vi "write time cell with column offset.vi"(5 "Column Relative?":bool, 7 "Header offset":i32, 8 "error in (no error)":errorcluster, 9 "time column offset":i32, 10 "start of last occupied row":cluster{"row":i32, "column":i32}, 11 "NI_report in":refnum<class "NI_report.lvclass">) -> (0 "error out":errorcluster, 3 "NI_report out":refnum<class "NI_report.lvclass">)   [LabVIEW 2016]
uses:
  <vilib>/Utility/NIReport.llb/NI_report.lvclass
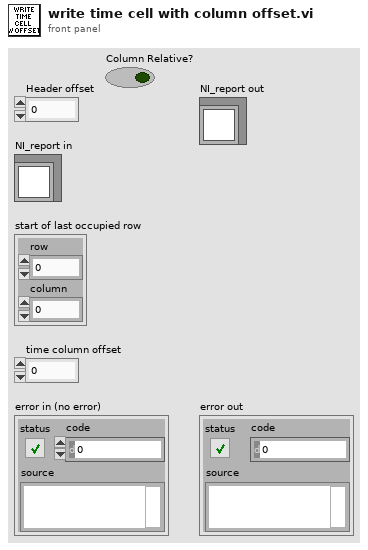
[diagram p1: front panel]
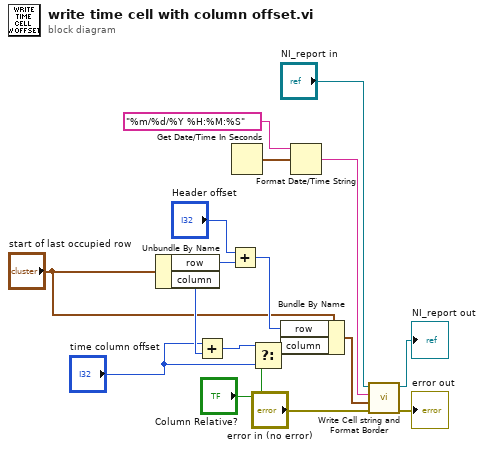
[diagram p0: block diagram]
diagram:
  n1 = Unbundle By Name("start of last occupied row") -> ("row"=w6:i32, "column"=w16:i32)
  n2 = Add(x="time column offset", y=w16) -> (x+y=w17:i32)
  n3 = Add(x="Header offset", y=w6) -> (x+y=w9:i32)
  n4 = Get Date/Time In Seconds() -> (seconds since 1Jan1904=w4:timestamp)
  n5 = Select(t=w17, s="Column Relative?", f="time column offset") -> (s? t:f=w3:i32)
  n6 = Bundle By Name(cluster="start of last occupied row", "row"=w9, "column"=w3) -> (w12:cluster{"row":i32, "column":i32})
  n7 = Format Date/Time String(time format string (%c)="%m/%d/%Y %H:%M:%S", seconds (now)=w4) -> (date/time string=w10:string)  [unwired: 1 in]
  n8 = call "Write Cell string and Format Border.vi"("error in (no error)"="error in (no error)", "output cluster"=w12, "input string"=w10, "NI_report in"="NI_report in") -> ("error out"=→"error out":errorcluster, "NI_report out"=→"NI_report out":refnum<class "NI_report.lvclass">)  [unwired: 6 in]
